vi "write_params.vi"(8 "error in (no error)":errorcluster, 10 "params":T1={"n_components"={"n_components_type"="None", "n_components_int"=0.0}, "kernel"="linear", "gamma"={"gamma_float"=0.0, "gamma_type"="None"}, "degree"=3.0, "coef0"=1.0, "alpha"=1.0, "fit_inverse_transform"=FALSE, "eigen_solver"="auto", "tol"=0.0, "max_iter"={"max_iter_type"="None", "max_iter_int"=0.0}, "remove_zero_eig"=FALSE, "random_state"=0.0, "copy_X"=TRUE, "n_jobs"=1.0}, 11 "KernelPCA in":refnum<class "KernelPCA.lvclass">) -> (0 "error out":errorcluster, 3 "KernelPCA out":refnum<class "KernelPCA.lvclass">)   [LabVIEW 2020, in "KernelPCA.lvclass"]
uses:
  KernelPCA.lvclass
  Controls/kernel_pca_params.ctl
  KernelPCA.lvclass/KernelPCA.ctl
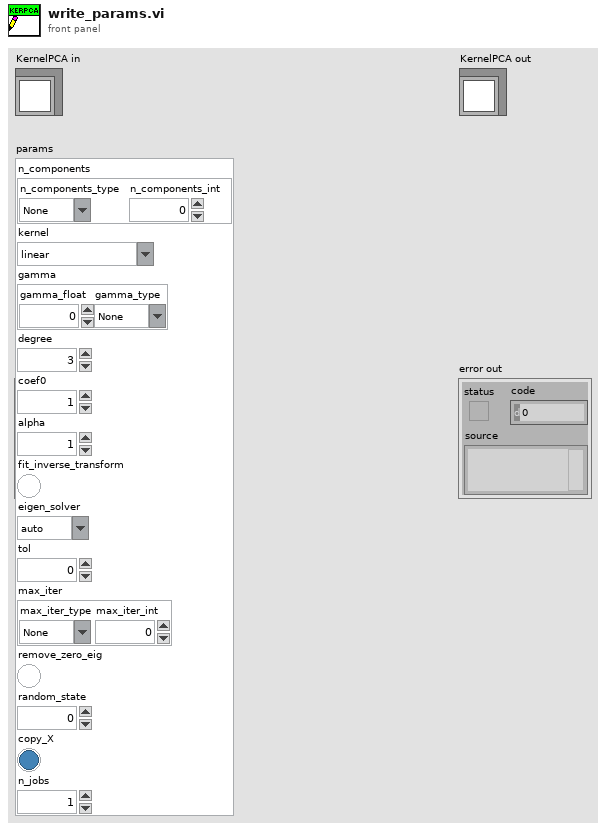
[diagram p1: front panel]
types:
  T1 = typedef "kernel_pca_params.ctl" = cluster{"n_components":cluster{"n_components_type":string, "n_components_int":dbl}, "kernel":string, "gamma":cluster{"gamma_float":dbl, "gamma_type":string}, "degree":dbl, "coef0":dbl, "alpha":dbl, "fit_inverse_transform":bool, "eigen_solver":string, "tol":dbl, "max_iter":cluster{"max_iter_type":string, "max_iter_int":dbl}, "remove_zero_eig":bool, "random_state":dbl, "copy_X":bool, "n_jobs":dbl}
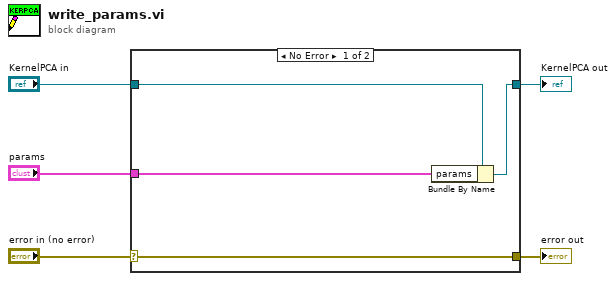
[diagram p0: block diagram]
diagram:
  n1 = case shown="No Error" "error in (no error)" {
    selector: "error in (no error)" -> [w9 w10]
    tunnel: [w9 w10] -> w4
    tunnel: [w7 w11] -> w2
    tunnel: "KernelPCA in" -> [w8 w11]
    tunnel: "params" -> [w6 _]
    frame No Error {
      n2 = Bundle By Name(cluster=w8, "params"=w6) -> (w7:refnum<class "KernelPCA.lvclass">)
    }
    frame Error {
    }
  }
  "error out" <- w4
  "KernelPCA out" <- w2
